vi "Modify Recipe Value.vi"(8 "error in (no error)":errorcluster, 9 "New Value":string, 10 "Key":string, 11 "Test Recipe in":refnum<class "Test Recipe.lvclass">) -> (0 "error out":errorcluster, 3 "Test Recipe out":refnum<class "Test Recipe.lvclass">)   [LabVIEW 2017, in "Test Recipe.lvlib" / "Test Recipe.lvclass"]
doc: "Programmtically updates a key/value pair in a recipe file and re-loads the recipe into memory to use the new file."
uses:
  Test Recipe.lvclass
  Test Recipe.lvclass/Test Recipe.ctl
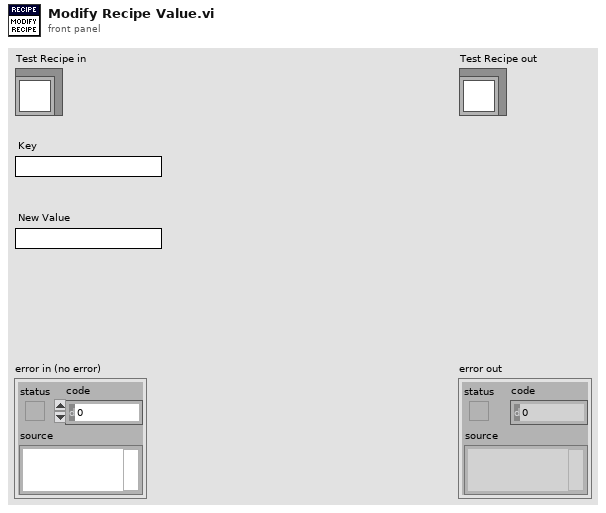
[diagram p1: front panel]
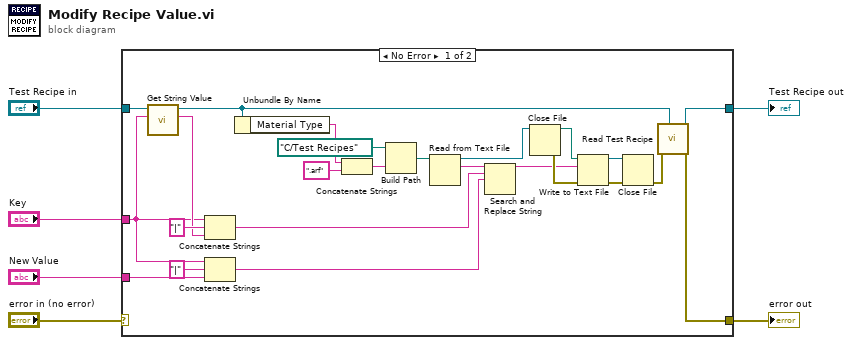
[diagram p0: block diagram]
diagram:
  n1 = case shown="No Error" "error in (no error)" {
    selector: "error in (no error)" -> [_ w32]
    tunnel: [w11 w32] -> w5
    tunnel: [w13 w31] -> w3
    tunnel: "Test Recipe in" -> [w24 w31]
    tunnel: "Key" -> [w19 _]
    tunnel: "New Value" -> [w20 _]
    frame No Error {
      n2 = call "Get String Value.vi"("Name"=w19, "Test Recipe in"=w24) -> ("Value"=w22:string, "Test Recipe out"=w8:refnum<class "Test Recipe.lvclass">)  [unwired: 6 in, 2 out]
      n3 = Concatenate Strings(w19, "|" ("string"), w22) -> (w18:string)
      n4 = Concatenate Strings(w19, "|" ("string"), w20) -> (w17:string)
      n5 = Unbundle By Name(w8) -> ("Material Type"=w7:string)
      n6 = Concatenate Strings(w7, ".arf" ("string")) -> (w28:string)
      n7 = Build Path(base path=path "C:/Test Recipes", name or relative path=w28) -> (appended path=w26:path)
      n8 = Read from Text File(file (use dialog)=w26) -> (refnum out=w10:refnum<file>, text=w25:string)  [unwired: 3 in, 2 out]
      n9 = Search and Replace String(input string=w25, search string=w18, replace string=w17) -> (result string=w16:string)  [unwired: 5 in, 3 out]
      n10 = Close File(refnum=w10) -> (path=w9:path, error out=w30:errorcluster)  [unwired: 1 in]
      n11 = Write to Text File(file (use dialog)=w9, text=w16, error in=w30) -> (refnum out=w15:refnum<file>, error out=w14:errorcluster)  [unwired: 1 in, 1 out]
      n12 = Close File(refnum=w15, error in=w14) -> (error out=w12:errorcluster)  [unwired: 1 out]
      n13 = call "Read Test Recipe.vi"("Test Recipe in"=w8, "error in (no error)"=w12) -> ("error out"=w11:errorcluster, "Test Recipe out"=w13:refnum<class "Test Recipe.lvclass">)  [unwired: 8 in]
    }
    frame Error {
    }
  }
  "error out" <- w5
  "Test Recipe out" <- w3
